vi "HPS-17000-PowerModule_GetAttributes.vi"(0 "reference in":refnum<class "HPS-17000-PowerModule.lvclass">, 5 "OnlyGetDvrReference(False)":bool, 11 "Error In":errorcluster) -> (4 "reference out":refnum<class "HPS-17000-PowerModule.lvclass">, 6 "Data":T1={"JSON Config Path"=path "", "Configuration"={"TSN NIC IP Address"="", "HPS17000 IP Addresses"=[], "HPS Topology"=enum."SINGLE", "Setpoint Stream Config"={"local address"="224.1.0.0", "receiver port"=61557}, "Measurement Array Size"=5000}, "GM ID"="", "HPS17000 Refs"=[], "connected"=FALSE, "reserved"=FALSE, "events"={"heartbeats events"=[], "faults events"=[], "network sync event"=[], "setpoint status event"=[]}, "nibatterycycler_grpc_Setpoint"={"voltage"=0.0, "current"=0.0, "min_power"=0.0, "max_power"=0.0, "resistance"=0.0}, "last timestamp"=0, "mode"=0, "range"={"Current Max (A)"=0.0, "Current Min (A)"=0.0, "Voltage Max (V)"=0.0, "Voltage Min (V)"=0.0}, "measurement array"=[]} {"mode" items=["NULL"=0, "CONSTANT VOLTAGE (V+R)"=1, "CONSTANT CURRENT (I)"=2, "V_VCC"=33, "V_VCC_R"=34, "V_VCC_RADJ"=35, "V_PI_IINT"=177, "INTERNAL RECIRCULATION (VCC)"=193, "INTERNAL RECIRCULATION (B2B)"=209, "VOLTAGE REFORMATION"=225]}, 10 "DataRef":refnum<data-value>, 15 "Error Out":errorcluster)   [LabVIEW 2023, in "HPS-17000-PowerModule.lvlib" / "HPS-17000-PowerModule.lvclass"]
uses:
  HPS-17000-PowerModule.lvclass
  protected/ObjectAttributes.ctl
  Configuration.ctl
  <vilib>/HPS-17000/Setpoint Stream Basic Config.ctl
  <instrlib>/HPS-17000/HPS-17000.lvclass
  <instrlib>/HPS-17000/Client Facing Datatypes/Multi-Cycler Events.ctl
  <instrlib>/HPS-17000/Client Facing Datatypes/Heartbeat Event Data.ctl
  <instrlib>/HPS-17000/Client Facing Datatypes/Faults Event Data.ctl
  <instrlib>/HPS-17000/Client Facing Datatypes/Network Sync Event Data.ctl
  <instrlib>/HPS-17000/Client Facing Datatypes/Setpoint Stream Status Data.ctl
  <vilib>/HPS-17000/nibatterycycler_grpc_Setpoint.ctl
  Mode.ctl
  builds/PowerModuleInterface/PowerModuleInterface.lvlibp/Classes/PowerModule_interface/Range.ctl
  builds/PowerModuleInterface/PowerModuleInterface.lvlibp/Classes/PowerModule_interface/Measurements.ctl
  HPS-17000-PowerModule.lvclass/HPS-17000-PowerModule.ctl
  <vilib>/HPS-17000/NI_BC_client.lvlib
  <vilib>/HPS-17000/Cycler.lvclass
  builds/PowerModuleInterface/PowerModuleInterface.lvlibp/Classes/PowerModule_interface/PowerModuleInterface.lvclass
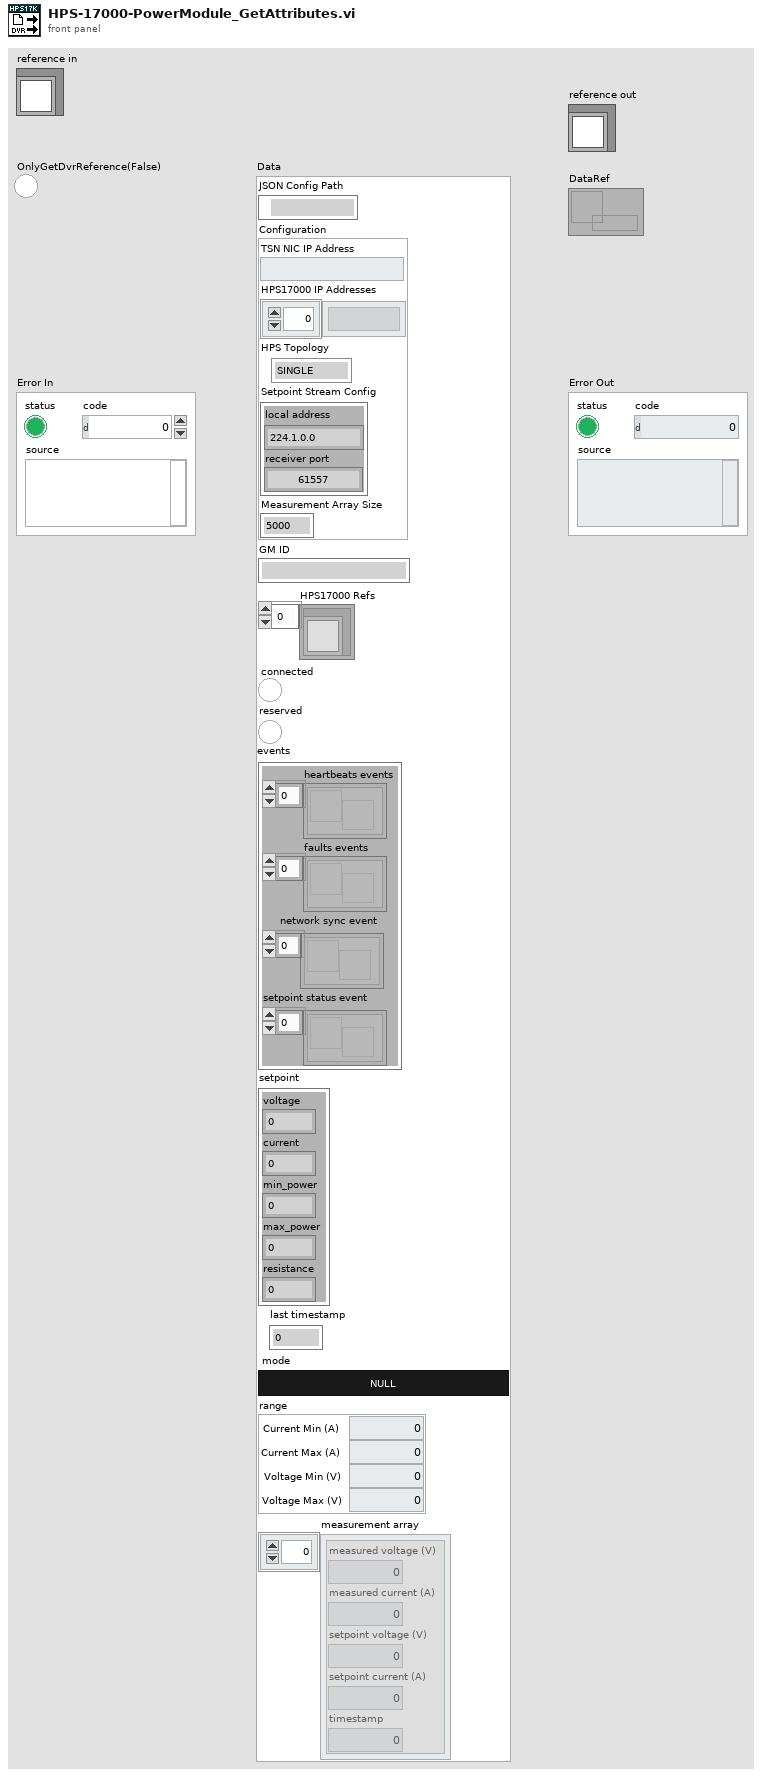
[diagram p1: front panel]
types:
  T1 = typedef "HPS-17000-PowerModule.lvlib/HPS-17000-PowerModule.lvclass/ObjectAttributes.ctl" = cluster{"JSON Config Path":path, "Configuration":T2, "GM ID":string, "HPS17000 Refs":refnum<class "HPS-17000.lvclass">[], "connected":bool, "reserved":bool, "events":T4, "nibatterycycler_grpc_Setpoint":T5, "last timestamp":i64, "mode":T6, "range":T7, "measurement array":T8[]}
  T2 = typedef "HPS-17000-PowerModule.lvlib/HPS-17000-PowerModule.lvclass/Configuration.ctl" = cluster{"TSN NIC IP Address":string, "HPS17000 IP Addresses":string[], "HPS Topology":enum16{"SINGLE", "MULTI"}, "Setpoint Stream Config":T3, "Measurement Array Size":i32}
  T3 = typedef "Cycler.lvclass/Setpoint Stream Basic Config.ctl" = cluster{"local address":string, "receiver port":u16}
  T4 = typedef "HPS-17000.lvclass/Multi-Cycler Events.ctl" = cluster{"heartbeats events":refnum<user-event>[], "faults events":refnum<user-event>[], "network sync event":refnum<user-event>[], "setpoint status event":refnum<user-event>[]}
  T5 = typedef "NI_BC_client.lvlib/nibatterycycler_grpc_Setpoint.ctl" = cluster{"voltage":sgl, "current":sgl, "min_power":sgl, "max_power":sgl, "resistance":sgl}
  T6 = typedef "HPS-17000-PowerModule.lvlib/HPS-17000-PowerModule.lvclass/Mode.ctl" = u16
  T7 = typedef "PowerModuleInterface.lvlibp/PowerModuleInterface.lvclass/Range.ctl" = cluster{"Current Max (A)":dbl, "Current Min (A)":dbl, "Voltage Max (V)":dbl, "Voltage Min (V)":dbl}
  T8 = typedef "PowerModuleInterface.lvlibp/PowerModuleInterface.lvclass/Measurements.ctl" = cluster{"measured voltage (V)":dbl, "measured current (A)":dbl, "setpoint voltage (V)":dbl, "setpoint current (A)":dbl, "timestamp":dbl}
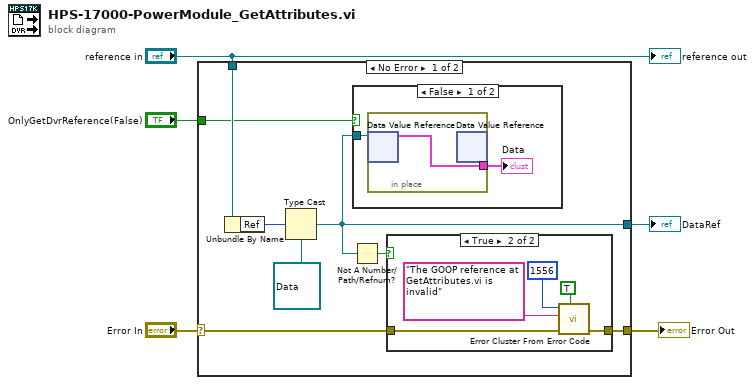
[diagram p0: block diagram]
diagram:
  n1 = case shown="No Error" "Error In" {
    selector: "Error In" -> [w7 w23]
    tunnel: "reference in" -> [w13 _]
    tunnel: [w12 _] -> w4
    tunnel: "OnlyGetDvrReference(False)" -> [w11 _]
    tunnel: [w6 w23] -> w1
    frame No Error {
      n2 = Unbundle By Name(w13) -> ("Ref"=w10:u32)
      n3 = Type Cast(type=refnum<data-value> refnum, x=w10) -> (*(type *) &x=w12:refnum<data-value>)
      n4 = Not A Number/Path/Refnum?(number/path/refnum=w12) -> (NaN/Path/Refnum?=w9:bool)
      n5 = case shown="False" w11 {
        tunnel: w12 -> [w21 _]
        frame False {
          n6 = in-place {
            in-place-border: [w22] -> w20
            n7 = in-place-dvr #1(w21) -> (w22:T1)  [unwired: 1 out]
            n8 = in-place-dvr #1() -> ()  [unwired: 1 in, 2 out]
          }
          "Data" <- w20
        }
        frame True {
        }
      }
      n9 = case shown="True" w9 {
        tunnel: w7 -> [w14 w17]
        tunnel: [w14 w16] -> w6
        frame False {
        }
        frame True {
          n10 = call <vilib>:"Error Cluster From Error Code.vi"("show call chain? (False)"=TRUE, "error in (no error)"=w17, "error message (\"\")"="The GOOP reference at GetAttributes.vi is invalid" ("source"), "error code (0)"=1556 ("code")) -> ("error out"=w16:errorcluster)  [unwired: 5 in]
        }
      }
    }
    frame Error {
    }
  }
  "DataRef" <- w4
  "Error Out" <- w1
  "reference out" <- "reference in"
